vi "Graham Scan Point Comparison Less Than.vi"(1 "B":T1, 2 "A":T1) -> (0 "A < B?":bool)   [LabVIEW 2018]
uses:
  Graham Scan Point.ctl
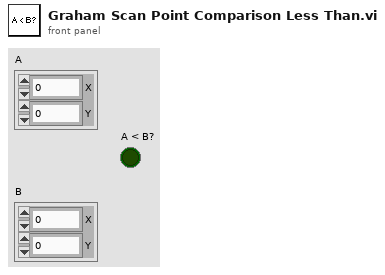
[diagram p1: front panel]
types:
  T1 = typedef "Graham Scan Point.ctl" = cluster{"X":i32, "Y":i32}
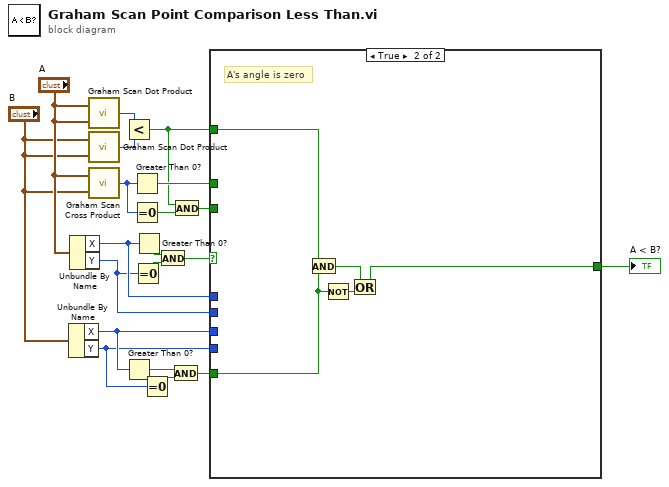
[diagram p0: block diagram]
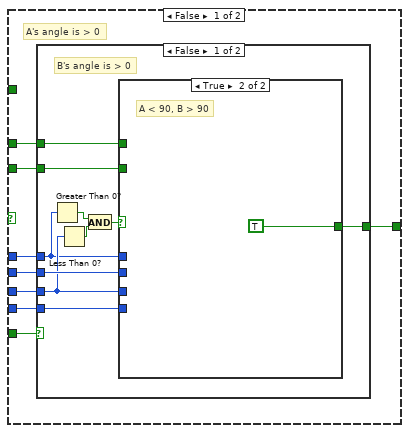
[diagram p2: hidden frame]
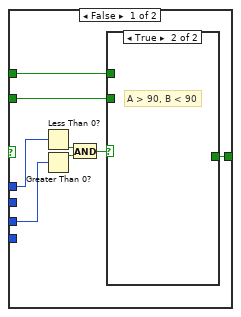
[diagram p3: hidden frame]
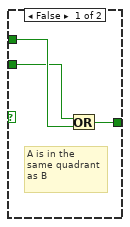
[diagram p4: hidden frame]
diagram:
  n1 = Unbundle By Name("B") -> ("X"=w14:i32, "Y"=w13:i32)
  n2 = Unbundle By Name("A") -> ("X"=w17:i32, "Y"=w16:i32)
  n3 = call "Graham Scan Dot Product.vi"("B"="A", "A"="A") -> ("C"=w6:i32)
  n4 = call "Graham Scan Dot Product.vi"("B"="B", "A"="B") -> ("C"=w5:i32)
  n5 = call "Graham Scan Cross Product.vi"("B"="B", "A"="A") -> ("C"=w4:i32)
  n6 = Less?(x=w6, y=w5) -> (x < y?=w2:bool)
  n7 = Greater Than 0?(x=w14) -> (x > 0?=w11:bool)
  n8 = Greater Than 0?(x=w4) -> (x > 0?=w9:bool)
  n9 = Equal To 0?(x=w4) -> (x = 0?=w3:bool)
  n10 = Equal To 0?(x=w16) -> (x = 0?=w20:bool)
  n11 = Greater Than 0?(x=w17) -> (x > 0?=w19:bool)
  n12 = Equal To 0?(x=w13) -> (x = 0?=w12:bool)
  n13 = And(x=w19, y=w20) -> (x .and. y?=w18:bool)
  n14 = And(x=w11, y=w12) -> (x .and. y?=w10:bool)
  n15 = And(x=w2, y=w3) -> (x .and. y?=w1:bool)
  n16 = case shown="True" w18 {
    tunnel: w17 -> [w26 _]
    tunnel: w16 -> [w27 _]
    tunnel: w14 -> [w25 _]
    tunnel: w13 -> [w24 _]
    tunnel: w9 -> [w23 _]
    tunnel: [w22 w52] -> w15
    tunnel: w10 -> [w28 w53]
    tunnel: w2 -> [_ w55]
    tunnel: w1 -> [w21 _]
    frame False {
      # "A's angle is > 0"
      n17 = case shown="False" w28 {
        tunnel: w27 -> [w35 _]
        tunnel: w26 -> [w32 _]
        tunnel: w25 -> [w33 _]
        tunnel: w24 -> [w34 _]
        tunnel: w23 -> [w30 _]
        tunnel: [w31 _] -> w22
        tunnel: w21 -> [w29 _]
        frame False {
          # "B's angle is > 0"
          n18 = Greater Than 0?(x=w32) -> (x > 0?=w38:bool)
          n19 = Less Than 0?(x=w33) -> (x < 0?=w37:bool)
          n20 = And(x=w38, y=w37) -> (x .and. y?=w36:bool)
          n21 = case shown="True" w36 {
            tunnel: w35 -> [_ _]
            tunnel: w34 -> [_ _]
            tunnel: w33 -> [w45 _]
            tunnel: w32 -> [w46 _]
            tunnel: [w40 TRUE] -> w31
            tunnel: w30 -> [w41 _]
            tunnel: w29 -> [w39 _]
            frame False {
              n22 = Less Than 0?(x=w46) -> (x < 0?=w44:bool)
              n23 = Greater Than 0?(x=w45) -> (x > 0?=w43:bool)
              n24 = And(x=w44, y=w43) -> (x .and. y?=w42:bool)
              n25 = case shown="True" w42 {
                tunnel: w41 -> [w49 _]
                tunnel: [w48 _] -> w40
                tunnel: w39 -> [w47 _]
                frame False {
                  # "A is in the\nsame quadrant\nas B"
                  n26 = Or(x=w47, y=w49) -> (x .or. y?=w48:bool)
                }
                frame True {
                  # "A > 90, B < 90"
                }
              }
            }
            frame True {
              # "A < 90, B > 90"
            }
          }
        }
        frame True {
          # "B's angle is zero"
        }
      }
    }
    frame True {
      # "A's angle is zero"
      n27 = And(x=w55, y=w53) -> (x .and. y?=w54:bool)
      n28 = Not(x=w53) -> (.not. x?=w51:bool)
      n29 = Or(x=w54, y=w51) -> (x .or. y?=w52:bool)
    }
  }
  "A < B?" <- w15
